vi "Read Listener Type.vi"(8 "error in (no error)":errorcluster, 11 "OAuthClient in":refnum<class "OAuthClient.lvclass">) -> (0 "error out":errorcluster, 2 "Listener Type":refnum<class "Connection.TCP.lvclass">, 3 "OAuthClient out":refnum<class "OAuthClient.lvclass">)   [LabVIEW 2020, in "OAuthClient.lvclass"]
uses:
  OAuthClient.lvclass
  <vilib>/LabVIEW Open Source Project/Connection/Connection.TCP/Connection.TCP.lvclass
  OAuthClient.lvclass/OAuthClient.ctl
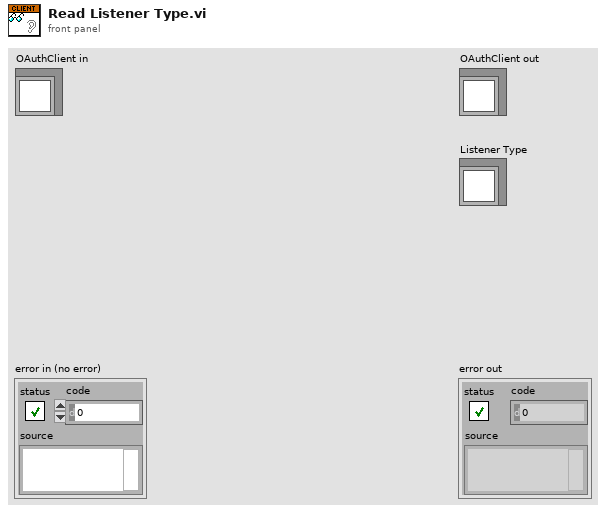
[diagram p1: front panel]
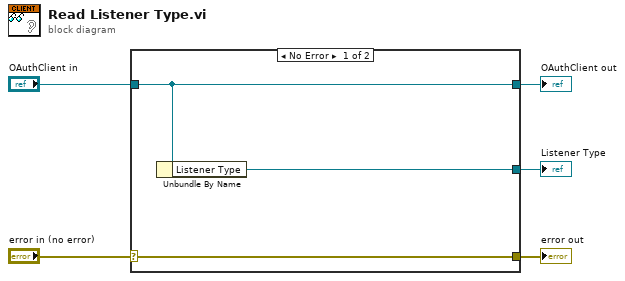
[diagram p0: block diagram]
diagram:
  n1 = case shown="No Error" "error in (no error)" {
    selector: "error in (no error)" -> [w8 w9]
    tunnel: [w8 w9] -> w4
    tunnel: [w7 w10] -> w2
    tunnel: "OAuthClient in" -> [w7 w10]
    tunnel: [w6 _] -> w1
    frame No Error {
      n2 = Unbundle By Name(w7) -> ("Listener Type"=w6:refnum<class "Connection.TCP.lvclass">)
    }
    frame Error {
    }
  }
  "error out" <- w4
  "OAuthClient out" <- w2
  "Listener Type" <- w1
